vi "cv_07_02.vi"() -> ()   [LabVIEW 2013]
panel:
  out "Square Root 2":dbl
  in  "Numeric 2":dbl
  out "Square Root":dbl
  in  "Numeric":dbl
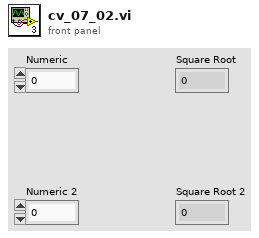
[diagram p1: front panel]
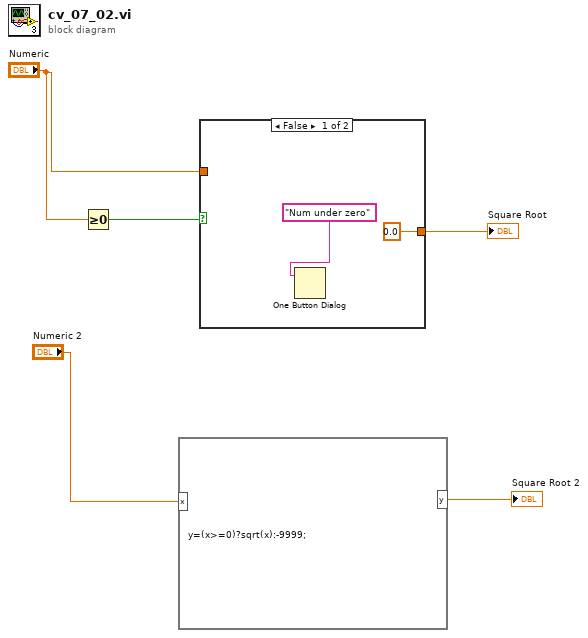
[diagram p0: block diagram]
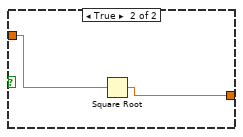
[diagram p2: hidden frame]
diagram:
  n1 = Greater Or Equal To 0?(x="Numeric") -> (x >= 0?=w5:bool)
  n2 = formula code="y=(x>=0)?sqrt(x):-9999;"("x"="Numeric 2") -> ("y"=→"Square Root 2":dbl)
  n3 = case shown="False" w5 {
    tunnel: "Numeric" -> [_ w9]
    tunnel: [0.0 w8] -> w3
    frame False {
      n4 = One Button Dialog(message="Num under zero") -> ()  [unwired: 1 in, 1 out]
    }
    frame True {
      n5 = Square Root(x=w9) -> (sqrt(x)=w8:dbl)
    }
  }
  "Square Root" <- w3
